vi "Instrument_dialog.vi"(2 "Ring":i32(ring) items=["Cpapir", "Simon", "Spectro", "SpiOMM", "PANO-II+CCD4Kx4K", "CCD4Kx4K", "PANO-I+EMCCD", "APP_SEPARATOR", "Modifier..."], 3 "Instrument liste":string[](array[string])) -> (0 "Index Output":i32, 1 "Output State":bool[](array[boolean]))   [LabVIEW 2010]
panel:
  in  "Confirm":bool
  in  "Probe_focus?":bool
  in  "use_exclusion?":bool
  in  "load_focus?":bool
  # "Choisissez les paramètres instrumentaux à être chargés ..."
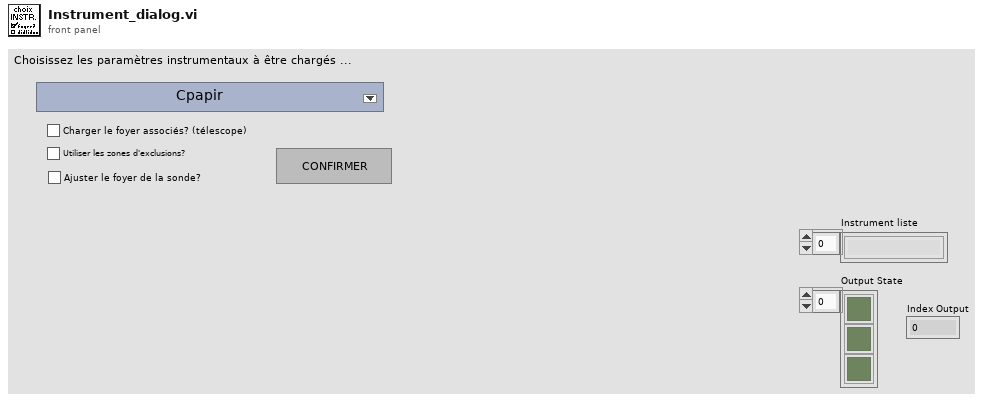
[diagram p1: front panel]
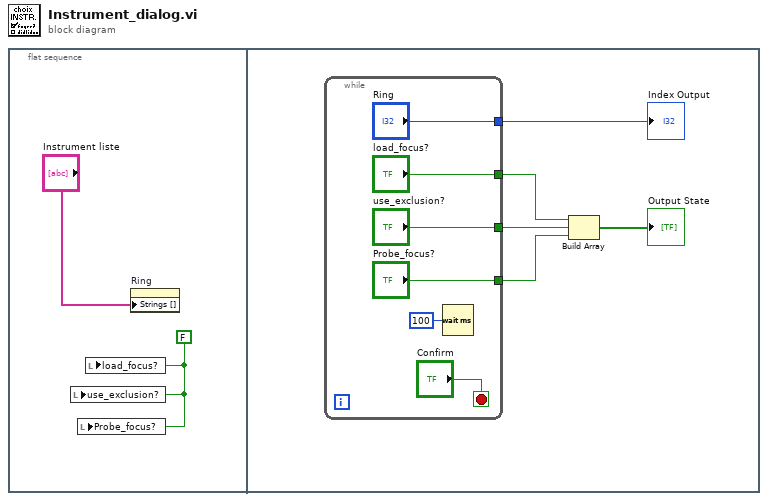
[diagram p0: block diagram]
diagram:
  n1 = flat-sequence {
    frame #0 {
      w1 = FALSE
      n2 = local write "use_exclusion?"(w1) -> ()
      n3 = local write "Probe_focus?"(w1) -> ()
      n4 = local write "load_focus?"(w1) -> ()
      n5 = property on="Ring" class="Ring (strict)"("Strings []"="Instrument liste") -> ()  [unwired: 2 in, 2 out]
    }
    frame #1 {
      n6 = while {
        tunnel: ["load_focus?"] -> w5
        tunnel: ["use_exclusion?"] -> w7
        tunnel: ["Probe_focus?"] -> w6
        tunnel: ["Ring"] -> w3
        stop <- "Confirm" stop-if-true
        n7 = Wait (ms)(milliseconds to wait=u32 100) -> ()  [unwired: 1 out]
      }
      "Index Output" <- w3
      n8 = Build Array(w5, w7, w6) -> (→"Output State":bool[])
    }
  }
